vi "Write promoted piece.vi"(10 "Piece (Queen)":T1=enum."Queen", 11 "Promotion in":refnum<class "Promotion.lvclass">) -> (3 "Promotion out":refnum<class "Promotion.lvclass">)   [LabVIEW 2016, in "Chesslib.lvlib" / "Promotion.lvclass"]
uses:
  Promotion.lvclass
  Promotion piece.ctl
  Promotion.lvclass/Promotion.ctl
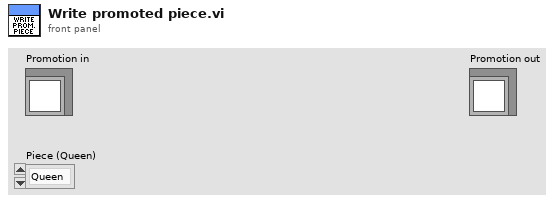
[diagram p1: front panel]
types:
  T1 = typedef "Chesslib.lvlib/Promotion.lvclass/Promotion piece.ctl" = enum16{"Bishop", "Knight", "Rook", "Queen"}
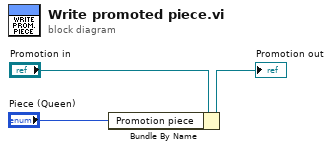
[diagram p0: block diagram]
diagram:
  n1 = Bundle By Name(cluster="Promotion in", "Promotion piece"="Piece (Queen)") -> (→"Promotion out":refnum<class "Promotion.lvclass">)
